vi "Tokenize  JSON String.vi"(10 "JSON String":string) -> (2 "Value Tokens":cluster{"Token Type":T1, "Token Value":string}[](array[cluster]))   [LabVIEW 2017, in "LVJSON.lvlib"]
uses:
  LVJSON.lvlib
  Token Types.ctl
panel:
  out "All Tokens":cluster{"Token Type":T1, "Token Value":string}[](array[cluster])
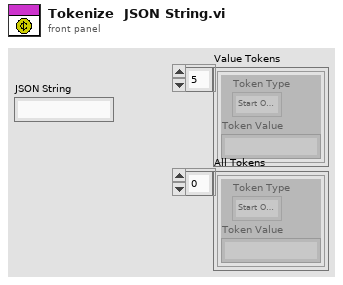
[diagram p1: front panel]
types:
  T1 = typedef "Token Types.ctl" = enum32{"Start Object", "End Object", "Start Array", "End Array", "Colon", "Comma", "Numeric", "true", "false", "null", "String"}
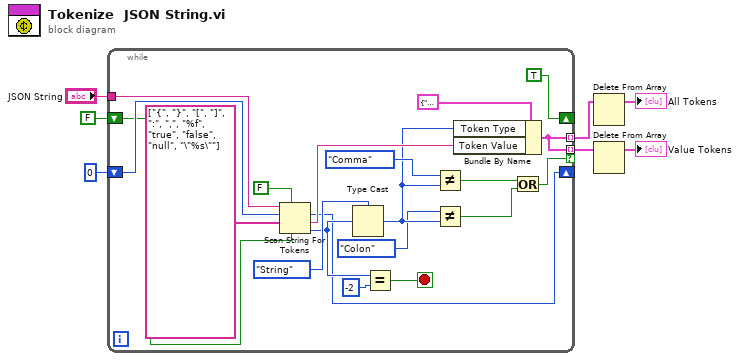
[diagram p0: block diagram]
diagram:
  n1 = while {
    tunnel: "JSON String" -> [w27]
    tunnel: [w13] -> w6 mode=indexing if=w11
    shift-right: [w16] -> _
    shift-left: 0 ("offset past token") -> [w17]
    shift-right: [TRUE] -> _
    shift-left: FALSE -> [w15]
    tunnel: [w13] -> w2 mode=indexing
    stop <- w23 stop-if-true
    n2 = Scan String For Tokens(4:w15, 5:FALSE ("allow empty tokens? (F)"), 7:string[] ["{", "}", "[", "]", ":", ",", "%f", "true", "false", "null", "\"%s\""] ("operators (none)"), 8:w17, 9:w27) -> (0:w20:i32, 1:w19:string, 2:w16:i32)  [unwired: 1 in, 1 out]
    n3 = Type Cast(type=Token_Types."String" ("Enum"), x=w20) -> (*(type *) &x=w9:T1)
    n4 = Equal?(x=w20, y=-2) -> (x = y?=w23:bool)
    n5 = Not Equal?(x=Token_Types."Comma", y=w9) -> (x != y?=w12:bool)
    n6 = Not Equal?(x=Token_Types."Colon", y=w9) -> (x != y?=w10:bool)
    n7 = Bundle By Name(cluster=cluster{"Token Type":T1, "Token Value":string} {"Token Type"=enum."String", "Token Value"=""} ("input cluster"), "Token Type"=w9, "Token Value"=w19) -> (w13:cluster{"Token Type":T1, "Token Value":string})
    n8 = Or(x=w12, y=w10) -> (x .or. y?=w11:bool)
  }
  n9 = Delete From Array(array=w2) -> (array with subset deleted=→"All Tokens":cluster{"Token Type":T1, "Token Value":string}[])  [unwired: 2 in, 1 out]
  n10 = Delete From Array(array=w6) -> (array with subset deleted=→"Value Tokens":cluster{"Token Type":T1, "Token Value":string}[])  [unwired: 2 in, 1 out]
